vi "Stop Core.vi"(10 "final error code":i32, 11 "Camera Simulator in":refnum<class "Camera Simulator.lvclass">) -> (3 "Camera Simulator out":refnum<class "Camera Simulator.lvclass">)   [LabVIEW 2020, in "Camera Simulator.lvlib" / "Camera Simulator.lvclass"]
doc: "(<B>Filename</B>: Actor Framework.lvlib:Actor.lvclass:Stop Core.vi)\n\nDefines what the actor does before it stops. Use the <B>final error code</B> input to determine whether the actor shut down in response to an error.\n\nBy default, this method does nothing. A descendant class may override it to define behavior, such as shutting down any processes the actor initiated in its override of the Actor Core method."
uses:
  Camera Simulator.lvclass
  <vilib>/ActorFramework/Time-Delayed Send Message/Time-Delay Override Options.ctl
  Camera Simulator.lvclass/Camera Simulator.ctl
  Camera Actor/Camera Actor/Camera Actor.lvclass
panel:
  out "error out":errorcluster
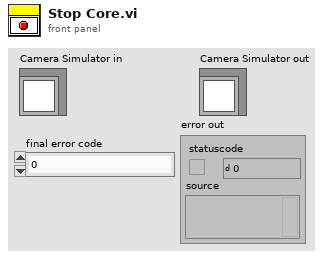
[diagram p1: front panel]
types:
  T1 = typedef "Time-Delay Override Options.ctl" = enum16{"Send next copy now", "Skip next scheduled copy", "Send next copy now and stop all further copies", "Stop all further copies"}
  T2 = typedef "IMAQ Image.ctl" = refnum<image>
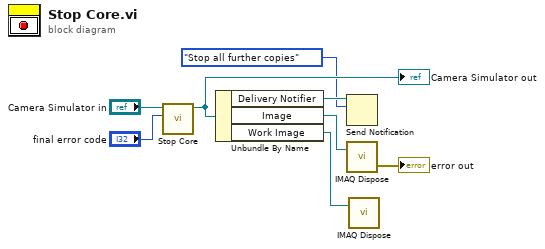
[diagram p0: block diagram]
diagram:
  n1 = call-parent "Stop Core.vi"("final error code"="final error code", "Camera Actor in"="Camera Simulator in") -> ("Camera Actor out"=w6:refnum<class "Camera Simulator.lvclass">)  [unwired: 9 in]
  "Camera Simulator out" <- w6
  n2 = Unbundle By Name(w6) -> ("Delivery Notifier"=w3:refnum<notifier>, "Image"=w5:T2, "Work Image"=w1:T2)
  n3 = Send Notification(notification=Time-Delay_Override_Options."Stop all further copies", notifier=w3) -> ()  [unwired: 1 in, 2 out]
  n4 = call "IMAQ Dispose"("Image"=w5) -> ("error out"=→"error out":errorcluster)  [unwired: 5 in]
  n5 = call "IMAQ Dispose"("Image"=w1) -> ()  [unwired: 5 in, 1 out]
